vi "RTS Get Point Location.vi"(8 "Error In":errorcluster, 11 "Full List Box Data":string[][](array[string])=[["System Date", "System Time", "Elapsed Time (sec)", "Elapsed Time (hrs)", "Voltage (V)", "RMS Current (Amps)", "Power (Watts)", "Watt Hours (Wh)", "Voltage Total Harmonic Distortion (%)", "Frequency (Hz)", "Apparent Power (VA)", "Power Factor", "TC 1", "TC 2", "TC 3", "TC 4", "TC 5", "TC 6", "TC 7", "TC 8", "TC 9", "TC 10", "TC 11", "TC 12", "TC 13", "TC 14", "TC 15", "TC 16", "TC 17", "TC 18", "TC 19", "TC 20", "TC 21", "TC 22", "TC 23", "TC 24", "TC 25", "TC 26", "TC 27", "TC 28", "TC 29", "TC 30", "AUX 1", "AUX 2", "CAL CL", "Room Setpoint Temperature", "Room Setpoint Humidity", "Room Temperature (°F)", "Room Humidity (%)", "Door Enable", "Room Setpoint Cool Temperature", "Room Setpoint Dehumidification Temperature", "Supply Temperature (°F)", "Cool Temperature (°F)", "Dehumidification Temperature (°F)", "Glycol Temperature (°F)", "Heat Rate (%)", "Steam Rate (%)", "Cool Rate (%)", "Dehumidification Rate (%)", "Room Status", "Room Dry P", "Room Dry I", "Room Humidity P", "Room Humidity I", "Room Heat P", "Room Heat I", "Room Cool Temperature P", "Room Cool Temperature I", "Room Dehumidification Temperature P", "Room Dehumidification Temperature I", "Voltage Setpoint 1", "60 Hz Power", "50 Hz Power", "120V Range", "240V Range", "Ground Line", "Ground Neutral", "Measure Ground Leakage Current", "Room OK", "S1 Freezer Relay", "S1 Cab Relay", "S1 Slide Relay", "Recording Data", "CVS Location", "Point Location"], ["01/26/2018", "13:16:19.991", "0.000000", "0.000000", "114.806053", "0.030120", "0.136762", "2048.346839", "3.400000", "59.984989", "3.457934", "1.000000", "-1.460000", "-1.480000", "-0.710000", "327.670000", "327.670000", "327.670000", "327.670000", "327.670000", "327.670000", "327.670000", "38.130000", "36.100000", "35.520000", "327.670000", "327.670000", "327.670000", "327.670000", "327.670000", "327.670000", "327.670000", "327.670000", "327.670000", "327.670000", "70.160000", "327.670000", "327.670000", "70.490000", "327.670000", "32767.000000", "32767.000000", "0.001000", "0.000000", "1.988000", "70.000000", "35.000000", "70.050000", "36.320000", "1.000000", "55.000000", "48.000000", "67.600000", "55.270000", "48.340000", "0.000000", "37.800000", "0.090000", "32.740000", "18.810000", "0.000000", "200.000000", "15000.000000", "400.000000", "15000.000000", "1000.000000", "2000.000000", "500.000000", "6000.000000", "500.000000", "6000.000000", "115.000000", "1.000000", "0.000000", "1.000000", "0.000000", "0.000000", "1.000000", "0.000000", "1.000000", "0.000000", "0.000000", "0.000000", "FALSE", "", "\\\\Evainlab01\\D$\\Hooks RTS\\Technology Lab\\NI-2010\\Trunk\\Refrigeration\\RTS\\Old System\\Point\\15P00183.pnt"]]) -> (0 "Error Out":errorcluster, 2 "Point File Name":string, 3 "Path":path)   [LabVIEW 2016]
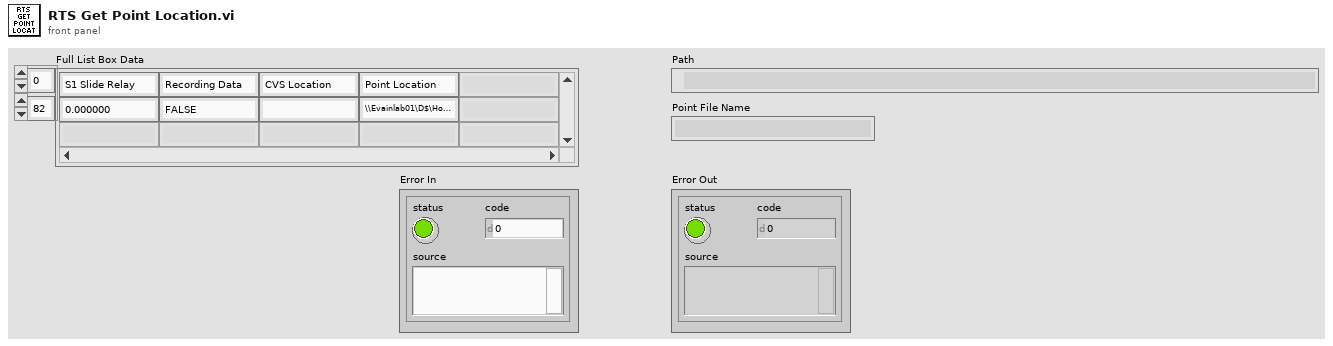
[diagram p1: front panel]
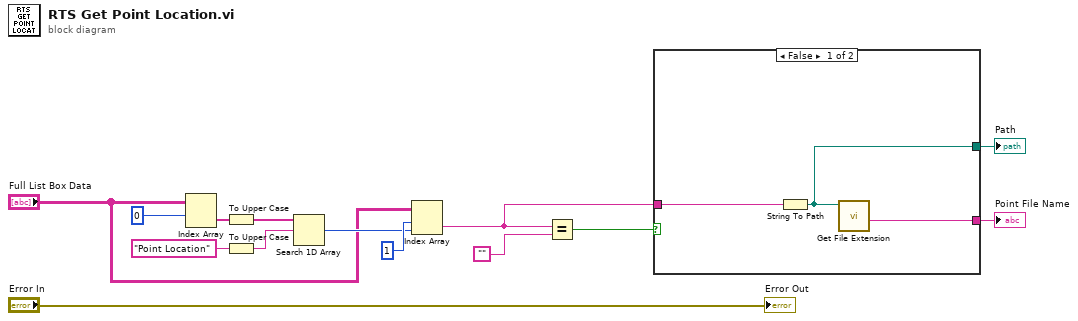
[diagram p0: block diagram]
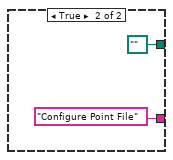
[diagram p2: hidden frame]
diagram:
  n1 = Index Array(array="Full List Box Data", index (row)=0) -> (element=w8:string[])  [unwired: 1 in]
  n2 = To Upper Case(1:w8) -> (0:w9:string[])
  n3 = To Upper Case(1:"Point Location" ("element")) -> (0:w11:string)
  n4 = Search 1D Array(1D array=w9, element=w11) -> (index of element=w13:i32)  [unwired: 1 in]
  n5 = Index Array(array="Full List Box Data", index (row)=1 ("disabled index (row)"), index (col)=w13) -> (element=w3:string)
  n6 = Equal?(x=w3, y="") -> (x = y?=w1:bool)
  n7 = case shown="False" w1 {
    tunnel: [w17 "Configure Point File" ("filename without extension")] -> w5
    tunnel: [w16 path ""] -> w4
    tunnel: w3 -> [w15 _]
    frame False {
      n8 = String To Path(string=w15) -> (path=w16:path)
      n9 = call <vilib>:"Get File Extension.vi"("file"=w16) -> ("filename without extension"=w17:string)  [unwired: 6 in, 4 out]
    }
    frame True {
    }
  }
  "Path" <- w4
  "Point File Name" <- w5
  "Error Out" <- "Error In"
